vi "PC_Main.vi"() -> ()   [LabVIEW 2018]
uses:
  <vilib>/Analysis/1siggen.llb/Ramp Pattern by Samples.vi
  <vilib>/Analysis/2dsp.llb/Power Spectrum (DBL).vi
  <vilib>/Utility/file.llb/Write Delimited Spreadsheet (string).vi
  <vilib>/Utility/file.llb/Write Delimited Spreadsheet (DBL).vi
  <vilib>/Analysis/NI_AALBase.lvlib
  <vilib>/Analysis/NI_AALPro.lvlib
panel:
  in  "delay (us)":dbl=8.4
  in  "base freq 3 (Hz)":fxp<+,18,17>=68000.0
  out "std phase 3":dbl caption="std(ph) (deg)" format="%0.2f"
  out "mean phase 3":dbl caption="phase (deg)" format="%0.2f"
  out "mean freq 3":dbl caption="f (Hz)" format="%0.2f"
  out "std freq 3":dbl caption="std(f) (Hz)" format="%0.2f"
  in  "f3 (kHz)":dbl=68.0
  in  "f2 (kHz)":dbl=32.0
  in  "f1 (kHz)":dbl=20.0
  in  "auto reset":bool
  out "ADC\nOverflow":bool
  out "Gain \ntoo high":bool
  in  "target ampl.":dbl=6.0 min=0.0 max=9.5
  in  "set auto gain":bool
  in  "Gain":fxp<+,20,8>=1.0
  in  "Pause Button":bool
  in  "refresh rate (Hz)":dbl=10.0
  out "std phase 2":dbl caption="std(ph) (deg)" format="%0.2f"
  out "mean phase 2":dbl caption="phase (deg)" format="%0.2f"
  out "mean freq 2":dbl caption="f (Hz)" format="%0.2f"
  out "std freq 2":dbl caption="std(f) (Hz)" format="%0.2f"
  in  "min std(f) (Hz)":dbl=10.0
  in  "filename":string="test"
  in  "Save":bool caption="Blank Button"
  out "saved as":path
  in  "Plot everything":bool=TRUE
  in  "store ratio":i16=4
  in  "base freq 2 (Hz)":fxp<+,18,17>=32000.0
  in  "Tab Control":T1(tab)=enum."Frequency"
  out "Spectrum":T2(graph)
  out "ADC in":cluster{dbl[], dbl[]}(graph)
  in  "scope idx":u8=1 min=1 max=3
  out "Phase PLL3":cluster{dbl[], dbl[]}(graph)
  out "Phase PLL1":cluster{dbl[], dbl[]}(graph)
  out "Phase PLL2":cluster{dbl[], dbl[]}(graph)
  out "Delta Frequency PLL1":cluster{dbl[], dbl[]}(graph)
  out "Delta Frequency PLL3":cluster{dbl[], dbl[]}(graph)
  out "Delta Frequency PLL2":cluster{dbl[], dbl[]}(graph)
  out "Frequency Spectrum PLL3":cluster{dbl[], dbl[]}(graph)
  out "Frequency Spectrum PLL1":cluster{dbl[], dbl[]}(graph)
  out "Frequency Spectrum PLL2":cluster{dbl[], dbl[]}(graph)
  in  "reset":bool
  in  "I gain":fxp<+,20,6>=6.5
  in  "P gain":fxp<+,14,14>=2000.0
  in  "base freq 1 (Hz)":fxp<+,18,17>=20000.0
  out "std phase 1":dbl caption="std(ph) (deg)" format="%0.2f"
  out "mean phase 1":dbl caption="phase (deg)" format="%0.2f"
  out "mean freq 1":dbl caption="f (Hz)" format="%0.2f"
  out "std freq 1":dbl caption="std(f) (Hz)" format="%0.2f"
  in  "Stop":bool
  in  "Stop RT":bool
  # "FPGA PLL - PC Main"
  # "Gain Settings"
  # "PLL Settings"
  # "Warnings"
  # "PLL 1"
  # "PLL 2"
  # "PLL 3"
  # "Live Scope"
  # "Save Data"
  # "t (ms)"
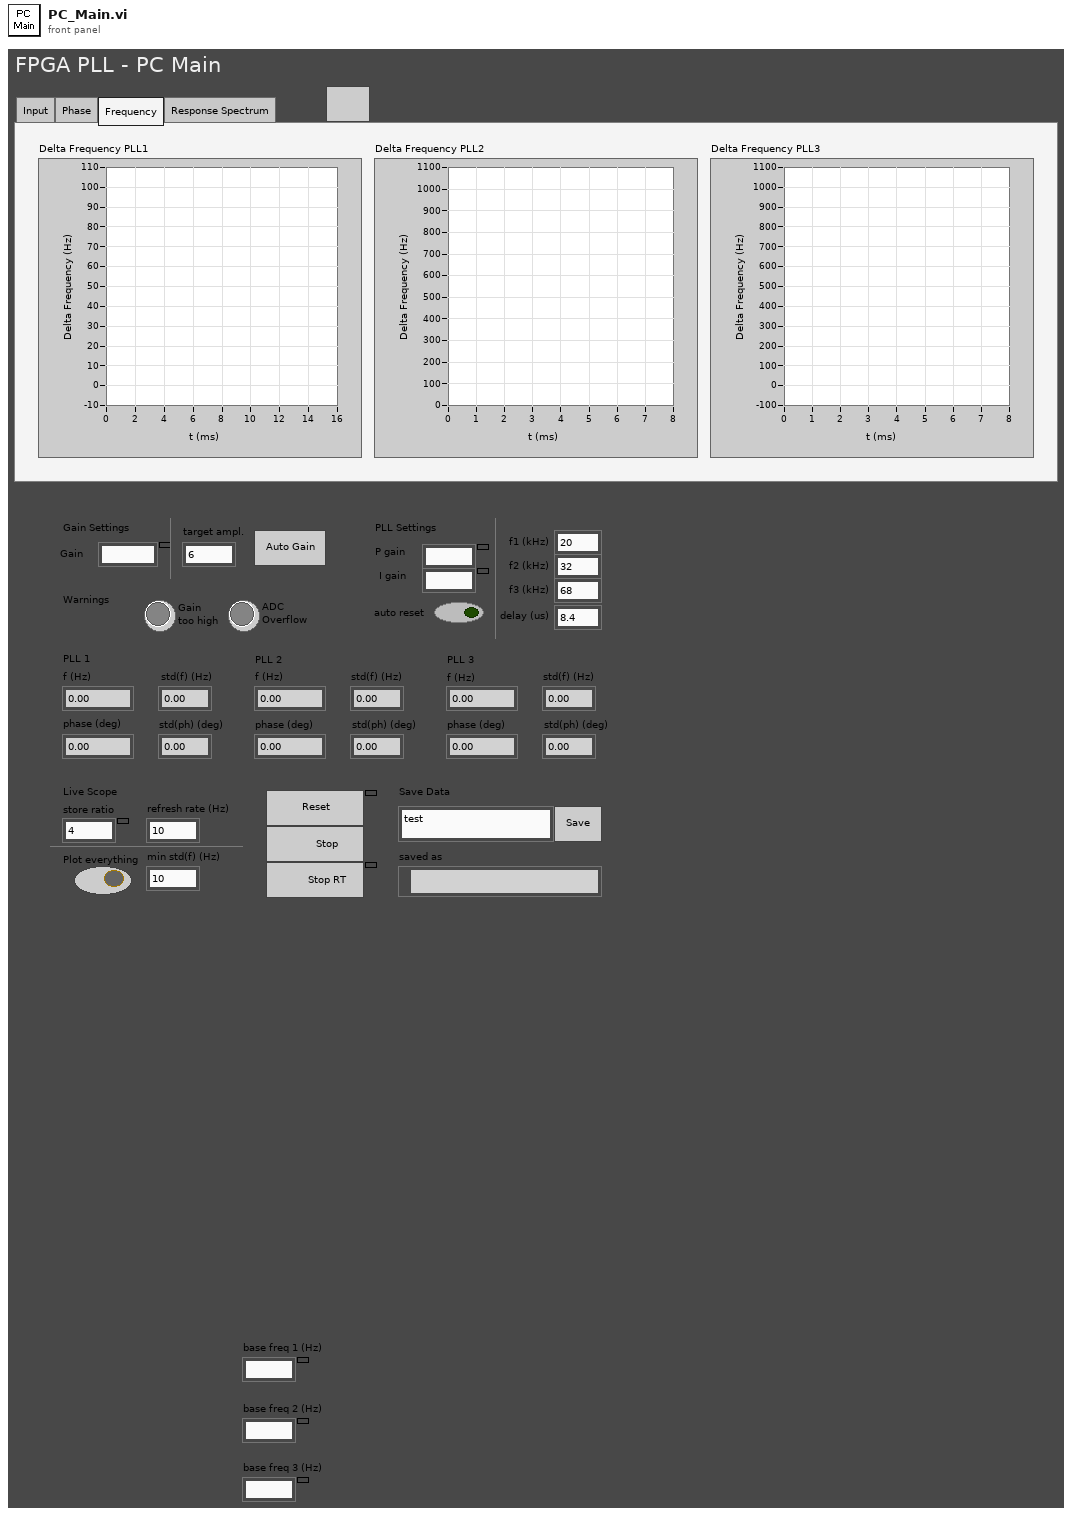
[diagram p1: front panel]
types:
  T1 = enum32{"Input", "Phase", "Frequency", "Response Spectrum"}
  T2 = cluster{"Ramp Pattern":dbl[], "Power Spectrum":dbl[]}[]
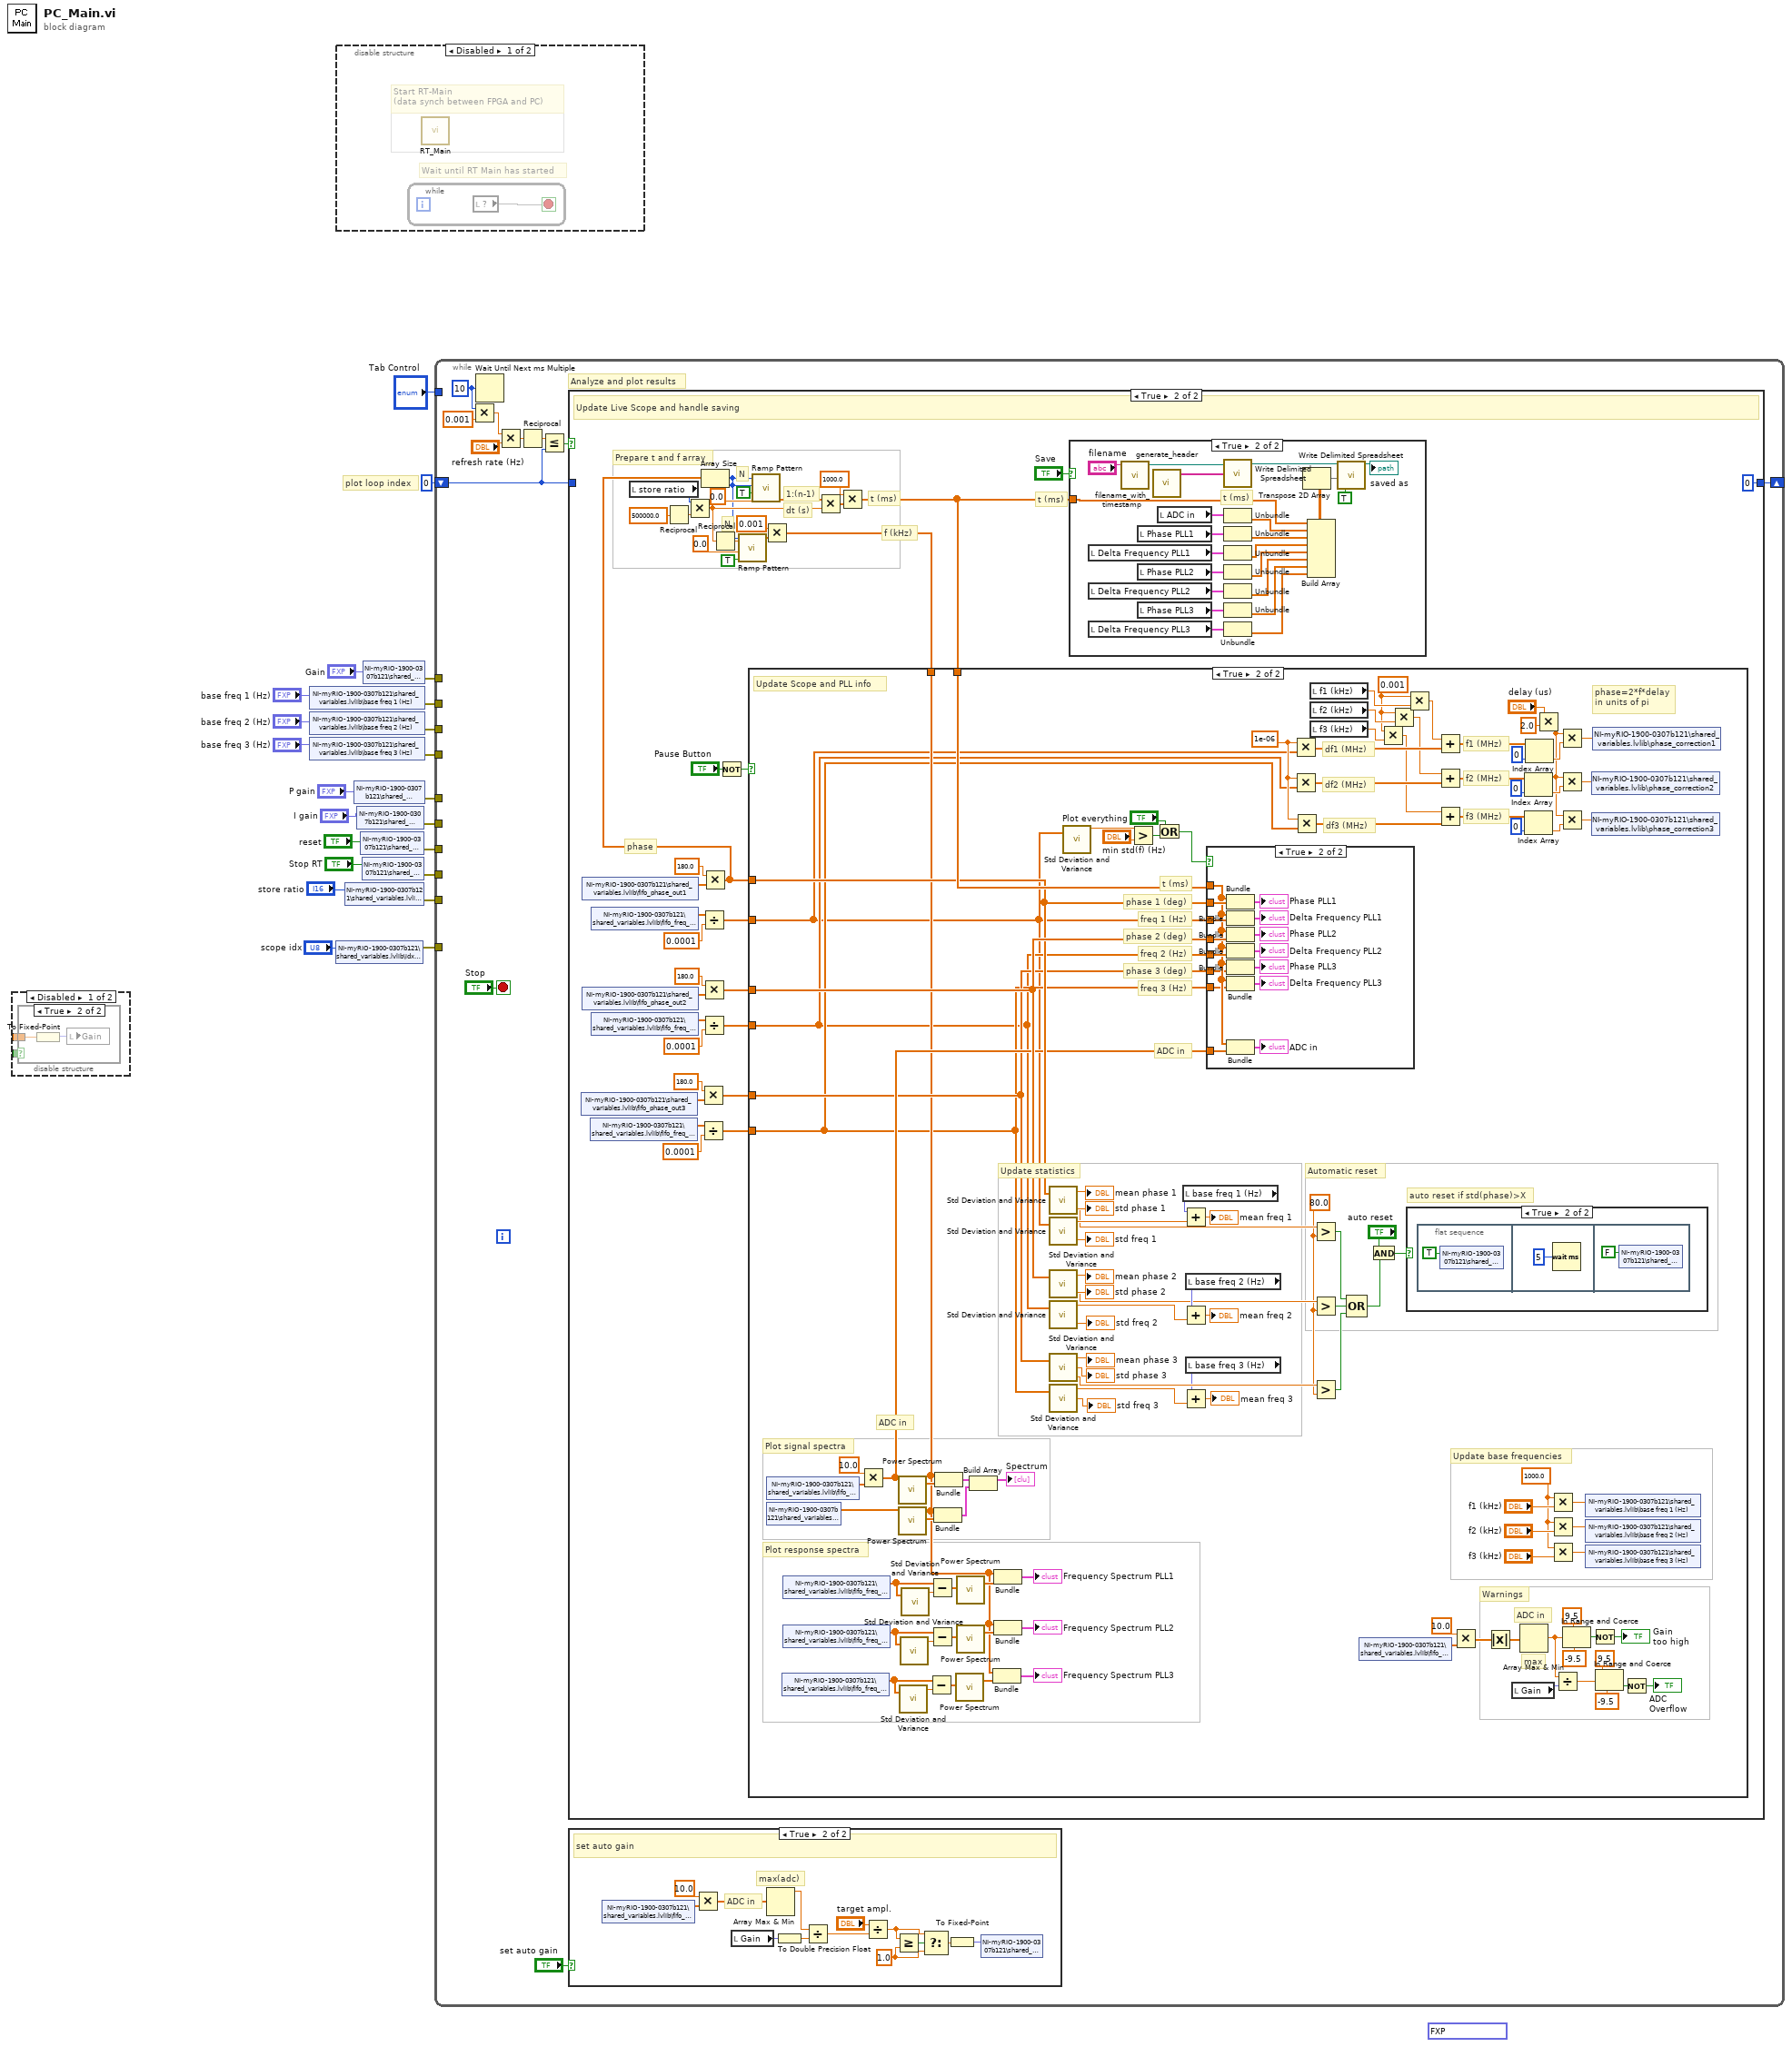
[diagram p0: block diagram]
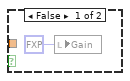
[diagram p2: hidden frame]
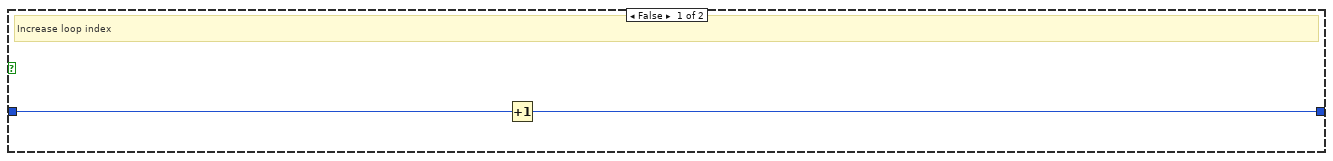
[diagram p5: hidden frame]
diagram:
  (unwired) fxp<+,12,0> 0.000244140625 ("y")
  # "plot loop index"
  n1 = disable-structure shown="Disabled" {
    disable-tunnel: _ -> [w24 _]
    disable-tunnel: _ -> [w23 _]
    frame Disabled {
      n2 = case shown="True" w23 {
        tunnel: w24 -> [_ w26]
        frame False {
          n3 = local write "Gain"(fxp<+,20,8> 1.0 ("Gain")) -> ()
        }
        frame True {
          n4 = To Fixed-Point(number=w26) -> (fixed-point=w27:fxp<+,20,8>)  [unwired: 1 in]
          n5 = local write "Gain"(w27) -> ()
        }
      }
    }
    frame Enabled {
    }
  }
  n6 = shared-variable "NI-myRIO-1900-0307b121\\shared_variables.lvlib\\base freq 1 (Hz)"("base freq 1 (Hz)") -> (error out=w20:errorcluster)  [unwired: 1 in]
  n7 = shared-variable "NI-myRIO-1900-0307b121\\shared_variables.lvlib\\base freq 2 (Hz)"("base freq 2 (Hz)") -> (error out=w5:errorcluster)  [unwired: 1 in]
  n8 = shared-variable "NI-myRIO-1900-0307b121\\shared_variables.lvlib\\base freq 3 (Hz)"("base freq 3 (Hz)") -> (error out=w4:errorcluster)  [unwired: 1 in]
  n9 = shared-variable "NI-myRIO-1900-0307b121\\shared_variables.lvlib\\idx_scope"("scope idx") -> (error out=w1:errorcluster)  [unwired: 1 in]
  n10 = disable-structure shown="Disabled" {
    frame Disabled {
      # "Wait until RT Main has started"
      # "Start RT-Main \n(data synch between FPGA and PC)"
      n11 = while {
        stop <- w28 stop-if-true
        n12 = local read item#-1() -> (w28)
      }
      n13 = call "RT_Main.vi"() -> ()  [unwired: 11 in, 1 out]
    }
    frame Enabled {
    }
  }
  n14 = shared-variable "NI-myRIO-1900-0307b121\\shared_variables.lvlib\\idx_pick"("store ratio") -> (error out=w12:errorcluster)  [unwired: 1 in]
  n15 = shared-variable "NI-myRIO-1900-0307b121\\shared_variables.lvlib\\P gain"("P gain") -> (error out=w19:errorcluster)  [unwired: 1 in]
  n16 = shared-variable "NI-myRIO-1900-0307b121\\shared_variables.lvlib\\I gain"("I gain") -> (error out=w18:errorcluster)  [unwired: 1 in]
  n17 = shared-variable "NI-myRIO-1900-0307b121\\shared_variables.lvlib\\reset"("reset") -> (error out=w16:errorcluster)  [unwired: 1 in]
  n18 = shared-variable "NI-myRIO-1900-0307b121\\shared_variables.lvlib\\stop"("Stop RT") -> (error out=w14:errorcluster)  [unwired: 1 in]
  n19 = shared-variable "NI-myRIO-1900-0307b121\\shared_variables.lvlib\\gain"("Gain") -> (error out=w7:errorcluster)  [unwired: 1 in]
  n20 = while {
    tunnel: w20 -> [_]
    tunnel: w19 -> [_]
    tunnel: w18 -> [_]
    tunnel: w16 -> [_]
    tunnel: w14 -> [_]
    tunnel: w12 -> [_]
    tunnel: "Tab Control" -> [_]
    shift-right: [w31] -> _
    shift-left: u32 0 -> [w30]
    tunnel: w7 -> [_]
    tunnel: w5 -> [_]
    tunnel: w4 -> [_]
    tunnel: w1 -> [_]
    stop <- "Stop" stop-if-true
    w35 = u32 10 ("millisecond multiple")
    # "Analyze and plot results"
    n21 = Multiply(x=w35, y=0.001 ("x")) -> (x*y=w34:dbl)
    n22 = Wait Until Next ms Multiple(millisecond multiple=w35) -> ()  [unwired: 1 out]
    n23 = Multiply(x=w34, y="refresh rate (Hz)") -> (x*y=w32:dbl)
    n24 = Reciprocal(x=w32) -> (1/x=w33:dbl)
    n25 = Less Or Equal?(x=w33, y=w30) -> (x <= y?=w39:bool)
    n26 = case shown="True" w39 {
      tunnel: w30 -> [w53 _]
      tunnel: [w54 u32 0] -> w31
      frame False {
        # "Increase loop index"
        n27 = Increment(x=w53) -> (x+1=w54:u32)
      }
      frame True {
        # "t (ms)"
        # "f (kHz)"
        # "t (ms)"
        # "phase"
        # "Prepare t and f array"
        # "N"
        # "N"
        # "dt (s)"
        # "1:(n-1)"
        # "Update Live Scope and handle saving"
        n28 = shared-variable "NI-myRIO-1900-0307b121\\shared_variables.lvlib\\fifo_phase_out3"() -> (w59:dbl[])  [unwired: 1 in, 1 out]
        n29 = shared-variable "NI-myRIO-1900-0307b121\\shared_variables.lvlib\\fifo_phase_out1"() -> (w92:dbl[])  [unwired: 1 in, 1 out]
        n30 = shared-variable "NI-myRIO-1900-0307b121\\shared_variables.lvlib\\fifo_phase_out2"() -> (w78:dbl[])  [unwired: 1 in, 1 out]
        n31 = shared-variable "NI-myRIO-1900-0307b121\\shared_variables.lvlib\\fifo_freq_out3"() -> (w60:dbl[])  [unwired: 1 in, 1 out]
        n32 = shared-variable "NI-myRIO-1900-0307b121\\shared_variables.lvlib\\fifo_freq_out1"() -> (w89:dbl[])  [unwired: 1 in, 1 out]
        n33 = shared-variable "NI-myRIO-1900-0307b121\\shared_variables.lvlib\\fifo_freq_out2"() -> (w61:dbl[])  [unwired: 1 in, 1 out]
        n34 = local read "store ratio"() -> (w87:i16)
        n35 = Reciprocal(x=500000.0) -> (1/x=w86:dbl)
        n36 = Multiply(x=w87, y=w86) -> (x*y=w70:dbl)
        n37 = Multiply(x=180.0, y=w59) -> (x*y=w57:dbl[])
        n38 = Divide(x=w60, y=0.0001 ("x")) -> (x/y=w56:dbl[])
        n39 = Divide(x=w89, y=0.0001 ("x")) -> (x/y=w75:dbl[])
        n40 = Multiply(x=180.0, y=w78) -> (x*y=w76:dbl[])
        n41 = Divide(x=w61, y=0.0001 ("x")) -> (x/y=w74:dbl[])
        n42 = Multiply(x=180.0, y=w92) -> (x*y=w62:dbl[])
        n43 = Array Size(array=w62) -> (size(s)=w68:i32)
        n44 = Reciprocal(x=w70) -> (1/x=w69:dbl)
        n45 = Not(x="Pause Button") -> (.not. x?=w63:bool)
        n46 = call-poly <vilib>:"Ramp Pattern.vi"("exclude end?"=TRUE, "start"=0.0, "end"=w69, "samples"=w68) -> ("Ramp Pattern"=w67:dbl[])  [unwired: 6 in, 1 out]
        n47 = call-poly <vilib>:"Ramp Pattern.vi"("exclude end?"=TRUE, "start"=0.0, "end"=w68, "samples"=w68) -> ("Ramp Pattern"=w77:dbl[])  [unwired: 6 in, 1 out]
        n48 = Multiply(x=0.001 ("start"), y=w67) -> (x*y=w65:dbl[])
        n49 = Multiply(x=w77, y=w70) -> (x*y=w81:dbl[])
        n50 = Multiply(x=1000.0, y=w81) -> (x*y=w73:dbl[])
        n51 = case shown="True" w63 {
          tunnel: w76 -> [_ w195]
          tunnel: w75 -> [_ w94]
          tunnel: w74 -> [_ w103]
          tunnel: w73 -> [_ w194]
          tunnel: w62 -> [_ w193]
          tunnel: w65 -> [_ w123]
          tunnel: w57 -> [_ w132]
          tunnel: w56 -> [_ w104]
          frame False {
          }
          frame True {
            w105 = 1e-06
            w99 = 0.001
            w147 = 1000.0 ("x")
            w133 = 80.0 ("y")
            # "df3 (MHz)"
            # "df2 (MHz)"
            # "df1 (MHz)"
            # "f3 (MHz)"
            # "phase=2*f*delay\nin units of pi"
            # "f1 (MHz)"
            # "f2 (MHz)"
            # "freq 3 (Hz)"
            # "phase 3 (deg)"
            # "Automatic reset"
            # "Update statistics"
            # "Update base frequencies"
            # "auto reset if std(phase)>X"
            # "Plot response spectra"
            # "Warnings"
            # "ADC in"
            # "max"
            # "Update Scope and PLL info"
            # "ADC in"
            # "Plot signal spectra"
            # "ADC in"
            # "freq 2 (Hz)"
            # "phase 2 (deg)"
            # "t (ms)"
            # "freq 1 (Hz)"
            # "phase 1 (deg)"
            n52 = shared-variable "NI-myRIO-1900-0307b121\\shared_variables.lvlib\\fifo_adc_in"() -> (w172:dbl[])  [unwired: 1 in, 1 out]
            n53 = shared-variable "NI-myRIO-1900-0307b121\\shared_variables.lvlib\\fifo_ref"() -> (w126:dbl[])  [unwired: 1 in, 1 out]
            n54 = shared-variable "NI-myRIO-1900-0307b121\\shared_variables.lvlib\\fifo_freq_out3"() -> (w144:dbl[])  [unwired: 1 in, 1 out]
            n55 = shared-variable "NI-myRIO-1900-0307b121\\shared_variables.lvlib\\fifo_freq_out1"() -> (w164:dbl[])  [unwired: 1 in, 1 out]
            n56 = shared-variable "NI-myRIO-1900-0307b121\\shared_variables.lvlib\\fifo_freq_out2"() -> (w161:dbl[])  [unwired: 1 in, 1 out]
            n57 = Multiply(x=10.0, y=w172) -> (x*y=w182:dbl[])
            n58 = call-poly <vilib>:"Power Spectrum.vi"("X"=w182) -> ("Power Spectrum"=w196:dbl[])  [unwired: 1 out]
            n59 = call-poly <vilib>:"Power Spectrum.vi"("X"=w126) -> ("Power Spectrum"=w125:dbl[])  [unwired: 1 out]
            n60 = call <vilib>:"Std Deviation and Variance.vi"("X"=w144) -> ("mean"=w143:dbl)  [unwired: 1 in, 2 out]
            n61 = call <vilib>:"Std Deviation and Variance.vi"("X"=w161) -> ("mean"=w162:dbl)  [unwired: 1 in, 2 out]
            n62 = call <vilib>:"Std Deviation and Variance.vi"("X"=w164) -> ("mean"=w165:dbl)  [unwired: 1 in, 2 out]
            n63 = Subtract(x=w144, y=w143) -> (x-y=w145:dbl[])
            n64 = Subtract(x=w164, y=w165) -> (x-y=w163:dbl[])
            n65 = Subtract(x=w161, y=w162) -> (x-y=w160:dbl[])
            n66 = Bundle(w123, "Power Spectrum"=w125) -> (w124:cluster{dbl[], "Power Spectrum":dbl[]})  [unwired: 1 in]
            n67 = Bundle(w123, "Power Spectrum"=w196) -> (w157:cluster{dbl[], "Power Spectrum":dbl[]})  [unwired: 1 in]
            n68 = call-poly <vilib>:"Power Spectrum.vi"("X"=w145) -> ("Power Spectrum"=w142:dbl[])  [unwired: 1 out]
            n69 = call-poly <vilib>:"Power Spectrum.vi"("X"=w163) -> ("Power Spectrum"=w167:dbl[])  [unwired: 1 out]
            n70 = call-poly <vilib>:"Power Spectrum.vi"("X"=w160) -> ("Power Spectrum"=w166:dbl[])  [unwired: 1 out]
            n71 = Build Array(w157, w124) -> (→"Spectrum":cluster{dbl[], "Power Spectrum":dbl[]}[])
            n72 = Bundle(w123, "Power Spectrum"=w142) -> (→"Frequency Spectrum PLL3":cluster{dbl[], "Power Spectrum":dbl[]})  [unwired: 1 in]
            n73 = Bundle(w123, "Power Spectrum"=w167) -> (→"Frequency Spectrum PLL1":cluster{dbl[], "Power Spectrum":dbl[]})  [unwired: 1 in]
            n74 = Bundle(w123, "Power Spectrum"=w166) -> (→"Frequency Spectrum PLL2":cluster{dbl[], "Power Spectrum":dbl[]})  [unwired: 1 in]
            n75 = call <vilib>:"Std Deviation and Variance.vi"("X"=w193) -> ("mean"=→"mean phase 1":dbl, "standard deviation"=→"std phase 1":dbl, "variance"=w158:dbl)  [unwired: 1 in]
            n76 = call <vilib>:"Std Deviation and Variance.vi"("X"=w94) -> ("mean"=w190:dbl, "standard deviation"=→"std freq 1":dbl)  [unwired: 1 in, 1 out]
            n77 = call <vilib>:"Std Deviation and Variance.vi"("X"=w195) -> ("mean"=→"mean phase 2":dbl, "standard deviation"=→"std phase 2":dbl, "variance"=w159:dbl)  [unwired: 1 in]
            n78 = call <vilib>:"Std Deviation and Variance.vi"("X"=w103) -> ("mean"=w187:dbl, "standard deviation"=→"std freq 2":dbl)  [unwired: 1 in, 1 out]
            n79 = call <vilib>:"Std Deviation and Variance.vi"("X"=w132) -> ("mean"=→"mean phase 3":dbl, "standard deviation"=→"std phase 3":dbl, "variance"=w140:dbl)  [unwired: 1 in]
            n80 = call <vilib>:"Std Deviation and Variance.vi"("X"=w104) -> ("mean"=w139:dbl, "standard deviation"=→"std freq 3":dbl)  [unwired: 1 in, 1 out]
            n81 = call <vilib>:"Std Deviation and Variance.vi"("X"=w94) -> ("standard deviation"=w203:dbl)  [unwired: 1 in, 2 out]
            n82 = Greater?(x=w203, y="min std(f) (Hz)") -> (0:w201:bool)
            n83 = Or(x="Plot everything", y=w201) -> (x .or. y?=w186:bool)
            n84 = local read "base freq 1 (Hz)"() -> (w191:fxp<+,18,17>)
            n85 = Add(x=w191, y=w190) -> (x+y=→"mean freq 1":dbl)
            n86 = local read "base freq 2 (Hz)"() -> (w189:fxp<+,18,17>)
            n87 = Add(x=w189, y=w187) -> (x+y=→"mean freq 2":dbl)
            n88 = local read "base freq 3 (Hz)"() -> (w138:fxp<+,18,17>)
            n89 = Add(x=w138, y=w139) -> (x+y=→"mean freq 3":dbl)
            n90 = case shown="True" w186 {
              tunnel: w193 -> [_ w223]
              tunnel: w94 -> [_ w222]
              tunnel: w194 -> [_ w213]
              tunnel: w195 -> [_ w219]
              tunnel: w103 -> [_ w218]
              tunnel: w182 -> [_ w216]
              tunnel: w104 -> [_ w212]
              tunnel: w132 -> [_ w211]
              frame False {
              }
              frame True {
                n91 = Bundle(w213, w223) -> (→"Phase PLL1":cluster{dbl[], dbl[]})  [unwired: 1 in]
                n92 = Bundle(w213, w222) -> (→"Delta Frequency PLL1":cluster{dbl[], dbl[]})  [unwired: 1 in]
                n93 = Bundle(w213, w219) -> (→"Phase PLL2":cluster{dbl[], dbl[]})  [unwired: 1 in]
                n94 = Bundle(w213, w218) -> (→"Delta Frequency PLL2":cluster{dbl[], dbl[]})  [unwired: 1 in]
                n95 = Bundle(w213, w211) -> (→"Phase PLL3":cluster{dbl[], dbl[]})  [unwired: 1 in]
                n96 = Bundle(w213, w212) -> (→"Delta Frequency PLL3":cluster{dbl[], dbl[]})  [unwired: 1 in]
                n97 = Bundle(w213, w216) -> (→"ADC in":cluster{dbl[], dbl[]})  [unwired: 1 in]
              }
            }
            n98 = Multiply(x=w105, y=w94) -> (x*y=w108:dbl[])
            n99 = Multiply(x=w105, y=w103) -> (x*y=w107:dbl[])
            n100 = Multiply(x=w105, y=w104) -> (x*y=w106:dbl[])
            n101 = local read "f1 (kHz)"() -> (w102:dbl)
            n102 = local read "f2 (kHz)"() -> (w101:dbl)
            n103 = local read "f3 (kHz)"() -> (w100:dbl)
            n104 = Greater?(x=w158, y=w133) -> (0:w130:bool)
            n105 = Greater?(x=w159, y=w133) -> (0:w128:bool)
            n106 = Greater?(x=w140, y=w133) -> (0:w129:bool)
            n107 = Compound Arithmetic op=OR(w130, w128, w129) -> (w127:bool)
            n108 = shared-variable "NI-myRIO-1900-0307b121\\shared_variables.lvlib\\fifo_adc_in"() -> (w171:dbl[])  [unwired: 1 in, 1 out]
            n109 = And(x="auto reset", y=w127) -> (x .and. y?=w153:bool)
            n110 = Multiply(x=w99, y=w100) -> (x*y=w98:dbl)
            n111 = Multiply(x=w99, y=w101) -> (x*y=w97:dbl)
            n112 = Multiply(x=w99, y=w102) -> (x*y=w96:dbl)
            n113 = case shown="True" w153 {
              frame False {
              }
              frame True {
                n114 = flat-sequence {
                  frame #0 {
                    n115 = shared-variable "NI-myRIO-1900-0307b121\\shared_variables.lvlib\\reset"(TRUE ("reset")) -> ()  [unwired: 1 in, 1 out]
                  }
                  frame #1 {
                    n116 = Wait (ms)(milliseconds to wait=u32 5) -> ()  [unwired: 1 out]
                  }
                  frame #2 {
                    n117 = shared-variable "NI-myRIO-1900-0307b121\\shared_variables.lvlib\\reset"(FALSE ("reset")) -> ()  [unwired: 1 in, 1 out]
                  }
                }
              }
            }
            n118 = Add(x=w96, y=w108) -> (x+y=w110:dbl[])
            n119 = Add(x=w97, y=w107) -> (x+y=w113:dbl[])
            n120 = Add(x=w98, y=w106) -> (x+y=w116:dbl[])
            n121 = Multiply(x=10.0, y=w171) -> (x*y=w155:dbl[])
            n122 = Absolute Value(x=w155) -> (abs(x)=w154:dbl[])
            n123 = local read "Gain"() -> (w178:fxp<+,20,8>)
            n124 = Array Max & Min(array=w154) -> (max value=w179:dbl)  [unwired: 3 out]
            n125 = Index Array(array=w113, index=0) -> (element=w119:dbl)
            n126 = Index Array(array=w116, index=0) -> (element=w115:dbl)
            n127 = Index Array(array=w110, index=0) -> (element=w122:dbl)
            n128 = Multiply(x="delay (us)", y=2.0) -> (x*y=w95:dbl)
            n129 = Multiply(x=w147, y="f1 (kHz)") -> (x*y=w152:dbl)
            n130 = Multiply(x=w147, y="f2 (kHz)") -> (x*y=w149:dbl)
            n131 = Multiply(x=w147, y="f3 (kHz)") -> (x*y=w148:dbl)
            n132 = Divide(x=w179, y=w178) -> (x/y=w176:dbl)
            n133 = Multiply(x=w95, y=w122) -> (x*y=w111:dbl)
            n134 = Multiply(x=w95, y=w119) -> (x*y=w117:dbl)
            n135 = Multiply(x=w95, y=w115) -> (x*y=w112:dbl)
            n136 = In Range and Coerce(upper limit=9.5, x=w179, lower limit=-9.5) -> (In Range?=w181:bool)  [unwired: 1 out]
            n137 = shared-variable "NI-myRIO-1900-0307b121\\shared_variables.lvlib\\base freq 1 (Hz)"(w152) -> ()  [unwired: 1 in, 1 out]
            n138 = shared-variable "NI-myRIO-1900-0307b121\\shared_variables.lvlib\\base freq 2 (Hz)"(w149) -> ()  [unwired: 1 in, 1 out]
            n139 = shared-variable "NI-myRIO-1900-0307b121\\shared_variables.lvlib\\base freq 3 (Hz)"(w148) -> ()  [unwired: 1 in, 1 out]
            n140 = Not(x=w181) -> (.not. x?=→"Gain \ntoo high":bool)
            n141 = shared-variable "NI-myRIO-1900-0307b121\\shared_variables.lvlib\\phase_correction2"(w117) -> ()  [unwired: 1 in, 1 out]
            n142 = shared-variable "NI-myRIO-1900-0307b121\\shared_variables.lvlib\\phase_correction3"(w112) -> ()  [unwired: 1 in, 1 out]
            n143 = shared-variable "NI-myRIO-1900-0307b121\\shared_variables.lvlib\\phase_correction1"(w111) -> ()  [unwired: 1 in, 1 out]
            n144 = In Range and Coerce(upper limit=9.5, x=w176, lower limit=-9.5) -> (In Range?=w173:bool)  [unwired: 1 out]
            n145 = Not(x=w173) -> (.not. x?=→"ADC\nOverflow":bool)
          }
        }
        n146 = case shown="True" "Save" {
          tunnel: w73 -> [_ w234]
          frame False {
          }
          frame True {
            # "t (ms)"
            n147 = local read "Delta Frequency PLL1"() -> (w238:cluster{dbl[], dbl[]})
            n148 = local read "Delta Frequency PLL2"() -> (w237:cluster{dbl[], dbl[]})
            n149 = local read "Delta Frequency PLL3"() -> (w228:cluster{dbl[], dbl[]})
            n150 = call "filename_with_timestamp.vi"("filename"="filename") -> ("filepath"=w230:path)  [unwired: 10 in]
            n151 = local read "Phase PLL1"() -> (w240:cluster{dbl[], dbl[]})
            n152 = local read "Phase PLL2"() -> (w239:cluster{dbl[], dbl[]})
            n153 = local read "Phase PLL3"() -> (w227:cluster{dbl[], dbl[]})
            n154 = call "generate_header.vi"() -> ("header\narray"=w231:string[])  [unwired: 11 in]
            n155 = local read "ADC in"() -> (w243:cluster{dbl[], dbl[]})
            n156 = call-poly <vilib>:"Write Delimited Spreadsheet.vi"("file path (dialog if empty)"=w230, "1D data"=w231) -> ("new file path (Not A Path if cancelled)"=w232:path)  [unwired: 12 in, 1 out]
            n157 = Unbundle(w243) -> (w242:dbl[])  [unwired: 1 out]
            n158 = Unbundle(w240) -> (w241:dbl[])  [unwired: 1 out]
            n159 = Unbundle(w238) -> (w236:dbl[])  [unwired: 1 out]
            n160 = Unbundle(w239) -> (w235:dbl[])  [unwired: 1 out]
            n161 = Unbundle(w237) -> (w233:dbl[])  [unwired: 1 out]
            n162 = Unbundle(w227) -> (w226:dbl[])  [unwired: 1 out]
            n163 = Unbundle(w228) -> (w225:dbl[])  [unwired: 1 out]
            n164 = Build Array(w234, w242, w241, w236, w235, w233, w226, w225) -> (w247:dbl[][])
            n165 = Transpose 2D Array(2D array=w247) -> (transposed array=w246:dbl[][])
            n166 = call-poly <vilib>:"Write Delimited Spreadsheet.vi"("file path (dialog if empty)"=w232, "2D data"=w246, "append to file? (new file:F)"=TRUE) -> ("new file path (Not A Path if cancelled)"=→"saved as":path)  [unwired: 11 in, 1 out]
          }
        }
      }
    }
    n167 = case shown="True" "set auto gain" {
      frame False {
      }
      frame True {
        w45 = 1.0 ("y")
        # "ADC in"
        # "max(adc)"
        # "set auto gain"
        n168 = shared-variable "NI-myRIO-1900-0307b121\\shared_variables.lvlib\\fifo_adc_in"() -> (w41:dbl[])  [unwired: 1 in, 1 out]
        n169 = Multiply(x=10.0, y=w41) -> (x*y=w48:dbl[])
        n170 = local read "Gain"() -> (w52:fxp<+,20,8>)
        n171 = Array Max & Min(array=w48) -> (max value=w51:dbl)  [unwired: 3 out]
        n172 = To Double Precision Float(number=w52) -> (double precision float=w50:dbl)
        n173 = Divide(x=w51, y=w50) -> (x/y=w44:dbl)
        n174 = Divide(x="target ampl.", y=w44) -> (x/y=w42:dbl)
        n175 = Greater Or Equal?(x=w42, y=w45) -> (x >= y?=w47:bool)
        n176 = Select(t=w42, s=w47, f=w45) -> (s? t:f=w46:dbl)
        n177 = To Fixed-Point(number=w46) -> (fixed-point=w40:fxp<+,20,8>)  [unwired: 1 in]
        n178 = shared-variable "NI-myRIO-1900-0307b121\\shared_variables.lvlib\\gain"(w40) -> ()  [unwired: 1 in, 1 out]
      }
    }
  }
